vi "Update Route Indicators.vi"(8 "error in":errorcluster, 9 "State in":bool, 10 "Name in":string, 11 "SwitchMatrix in":refnum<class "SwitchMatrix.lvclass">) -> (0 "error out":errorcluster, 1 "State out":bool, 2 "Name out":string, 3 "SwitchMatrix out":refnum<class "SwitchMatrix.lvclass">)   [LabVIEW 2019, in "SwitchMatrix.lvlib" / "SwitchMatrix.lvclass"]
uses:
  Library/SwitchMatrix.lvclass
  Library/SwitchMatrix.lvclass/SwitchMatrix.ctl
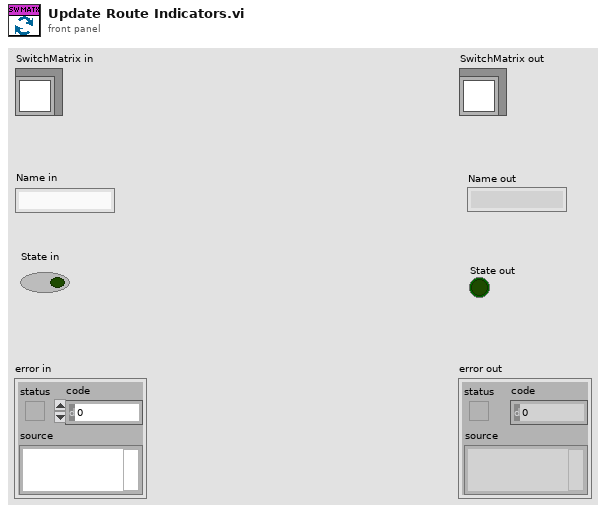
[diagram p1: front panel]
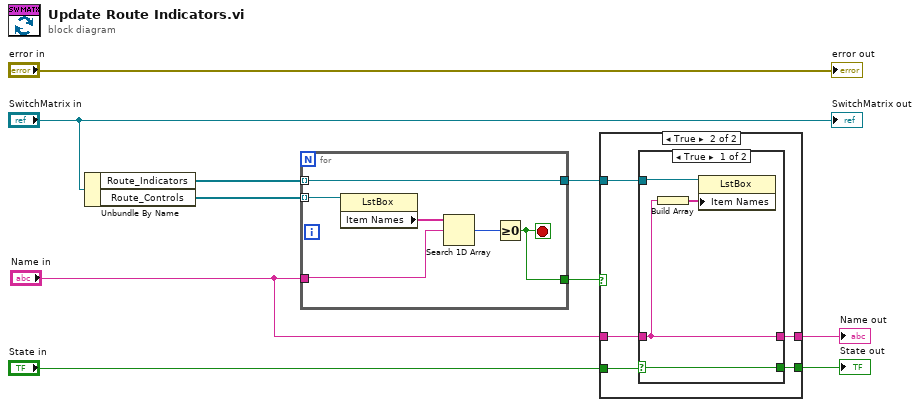
[diagram p0: block diagram]
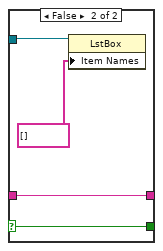
[diagram p3: hidden frame]
diagram:
  n1 = Unbundle By Name("SwitchMatrix in") -> ("Route_Indicators"=w8:refnum<vi>[], "Route_Controls"=w9:refnum<vi>[])
  n2 = for {
    tunnel: w9 -> [w15] mode=indexing
    tunnel: w8 -> [w16] mode=indexing
    tunnel: [w16] -> w4
    tunnel: "Name in" -> [w13]
    tunnel: [w11] -> w6
    stop <- w11 stop-if-true
    n3 = property class="LstBox"(reference=w15) -> ("Item Names"=w14:string[])  [unwired: 1 in, 2 out]
    n4 = Search 1D Array(1D array=w14, element=w13) -> (index of element=w12:i32)  [unwired: 1 in]
    n5 = Greater Or Equal To 0?(x=w12) -> (x >= 0?=w11:bool)
  }
  n6 = case shown="True" w6 {
    tunnel: "State in" -> [w17 w23]
    tunnel: w4 -> [_ w21]
    tunnel: "Name in" -> [w18 w22]
    tunnel: [w17 w20] -> w1
    tunnel: [w18 w19] -> w2
    frame False {
    }
    frame True {
      n7 = case shown="True" w23 {
        selector: w23 -> [w24 w29]
        tunnel: w22 -> [w25 w28]
        tunnel: w21 -> [w27 w31]
        tunnel: [w24 w29] -> w20
        tunnel: [w25 w28] -> w19
        frame True {
          n8 = Build Array(w25) -> (w26:string[])
          n9 = property class="LstBox"(reference=w27, "Item Names"=w26) -> ()  [unwired: 1 in, 2 out]
        }
        frame False {
          n10 = property class="LstBox"(reference=w31, "Item Names"=string[] []) -> ()  [unwired: 1 in, 2 out]
        }
      }
    }
  }
  "Name out" <- w2
  "State out" <- w1
  "error out" <- "error in"
  "SwitchMatrix out" <- "SwitchMatrix in"
